vi "comet_thermo_get_values_HTTP.vi"(8 "error in":errorcluster, 10 "timeout (5000)":i32=5000, 11 "IP":string) -> (0 "error out":errorcluster, 1 "p [hPa]":dbl, 2 "RH [%]":dbl, 3 "t [C]":dbl, 5 "p4":dbl)   [LabVIEW 2020]
uses:
  <vilib>/httpClient/LabVIEWHTTPClient.lvlib
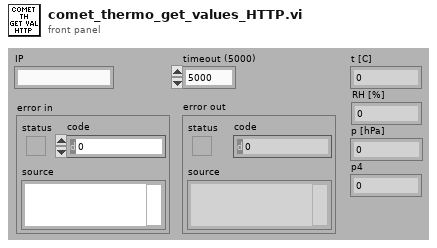
[diagram p1: front panel]
types:
  T1 = typedef "LabVIEWHTTPClient.lvlib/ClientHandle.ctl" = refnum<k1>
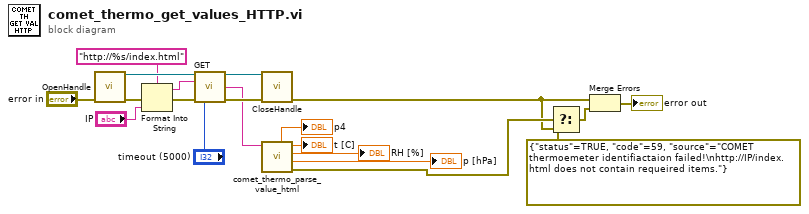
[diagram p0: block diagram]
diagram:
  n1 = call <vilib>:"OpenHandle.vi"("error in (no error)"="error in") -> ("client handle out"=w20:T1, "error out"=w17:errorcluster)  [unwired: 13 in]
  n2 = Format Into String(format string="http://%s/index.html", error in=w17, "IP") -> (resulting string=w15:string, error out=w18:errorcluster)  [unwired: 1 in]
  n3 = call <vilib>:"GET.vi"("client handle"=w20, "url"=w15, "error in (no error)"=w18, "timeout (10000)"="timeout (5000)") -> ("client handle out"=w12:T1, "body"=w10:string, "error out"=w13:errorcluster)  [unwired: 8 in, 1 out]
  n4 = call <vilib>:"CloseHandle.vi"("client handle"=w12, "error in (no error)"=w13) -> ("error out"=w1:errorcluster)  [unwired: 13 in]
  n5 = call "comet_thermo_parse_value_html.vi"("String"=w10) -> ("error out"=w5:errorcluster, "p [hPa]"=→"p [hPa]":dbl, "RH [%]"=→"RH [%]":dbl, "t [C]"=→"t [C]":dbl, "p4"=→"p4":dbl)  [unwired: 6 in]
  n6 = Select(t=errorcluster {"status"=TRUE, "code"=59, "source"="COMET thermoemeter identifiactaion failed!\nhttp://IP/index.html does not contain requeired items."} ("f"), s=w5, f=w1) -> (s? t:f=w4:errorcluster)
  n7 = Merge Errors(w1, w4) -> (→"error out":errorcluster)
